vi "Copy Slot.vi"(8 "error in":errorcluster, 10 "destination slot ref in":T1 format="%.0x", 11 "source slot ref in":T1 format="%.0x") -> (0 "error out":errorcluster, 2 "destination slot ref out":T1 format="%.0x", 3 "source slot ref out":T1 format="%.0x")   [LabVIEW 2019, in "Scan Engine Scripting.lvlib"]
doc: "Copies the slot configuration to another slot. Use this VI to quickly duplicate modules into other slots."
uses:
  Scan Engine Scripting.lvlib
  Includes/Modules.lvlibp/RSI Module/RSI Module.lvclass
  <vilib>/NI VeriStand/Custom Device API/Custom Device Item Ref.ctl
  <vilib>/NI VeriStand/Custom Device API/Custom Device API.lvlib
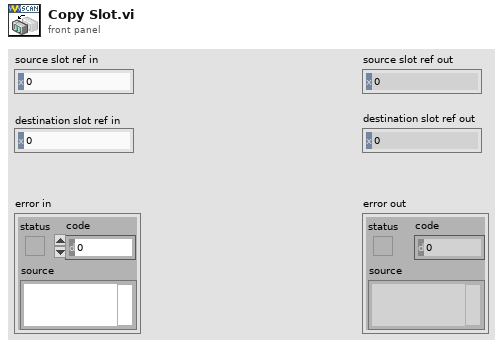
[diagram p1: front panel]
types:
  T1 = typedef "Custom Device API.lvlib/Custom Device Item Ref.ctl" = u64
  T2 = typedef "Modules.lvlibp/Custom Device API.lvlib/Custom Device Item Ref.ctl" = u64
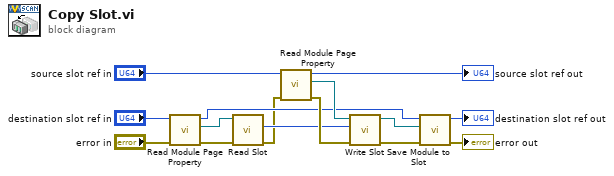
[diagram p0: block diagram]
diagram:
  n1 = call "Read Module Page Property.vi"("error in (no error)"="error in", "Node Ptr In"="destination slot ref in") -> ("error out"=w4:errorcluster, "RSI Module"=w13:refnum<class "RSI Module.lvclass">, "Node Ptr Out"=w3:T2)  [unwired: 7 in]
  n2 = call "Read Slot.vi"("error in (no error)"=w4, "RSI Module in"=w13) -> ("error out"=w1:errorcluster, "Slot"=w10:u32)  [unwired: 7 in, 1 out]
  n3 = call "Read Module Page Property.vi"("error in (no error)"=w1, "Node Ptr In"="source slot ref in") -> ("error out"=w11:errorcluster, "RSI Module"=w9:refnum<class "RSI Module.lvclass">, "Node Ptr Out"=→"source slot ref out":T2)  [unwired: 7 in]
  n4 = call "Write Slot.vi"("error in (no error)"=w11, "Slot"=w10, "RSI Module in"=w9) -> ("error out"=w5:errorcluster, "RSI Module out"=w12:refnum<class "RSI Module.lvclass">)  [unwired: 7 in]
  n5 = call "Save Module to Slot.vi"("error in"=w5, "RSI module in"=w12, "slot ref in"=w3) -> ("error out"=→"error out":errorcluster, "slot ref out"=→"destination slot ref out":T2)  [unwired: 6 in, 1 out]
